vi "DB Driver Main.vi"(0 "Table /DBName/Query":string="KMP", 1 "Option":T1, 2 "Database Name":string="MISPLDBSK06", 5 "Column Names":string[](array[string]), 9 "DB Connection Details":cluster{"UserID":string, "Password":string}={"UserID"="sa", "Password"="12345"}, 11 "error in":errorcluster, 12 "Where":string, 13 "Workstation ID/ Pc Name":string="MISPLDBSK06", 14 "Order By":string) -> (3 "Record Affected":i32, 4 "ADODB._Connection":refnum<k7>, 6 "Selected Data":string[][](array[string]), 10 "element":string, 15 "error out":errorcluster)   [LabVIEW 2017]
uses:
  DB Driver Main Options.ctl
panel:
  out "No.of Row":i32
  # "Output"
  # "Input"
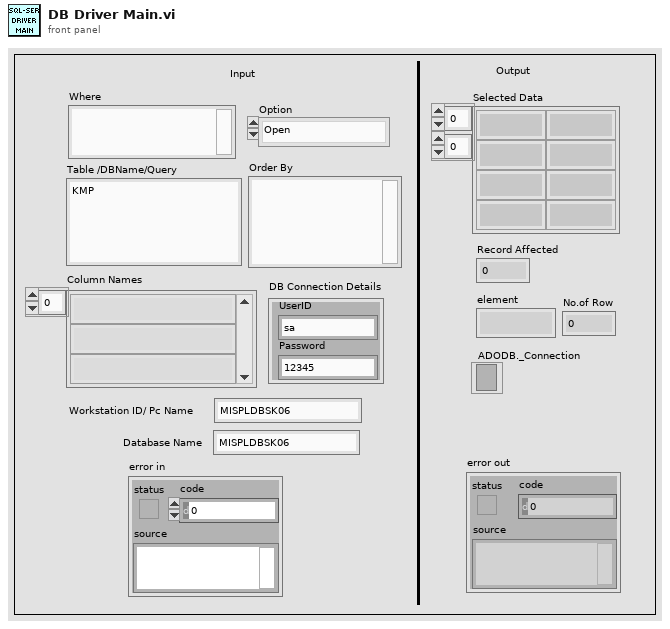
[diagram p1: front panel]
types:
  T1 = typedef "DB Driver Main Options.ctl" = enum16{"Open", "RefOut", "Select", "Execute", "Update", "Insert 2D", "Insert OrUpdate", "Close"}
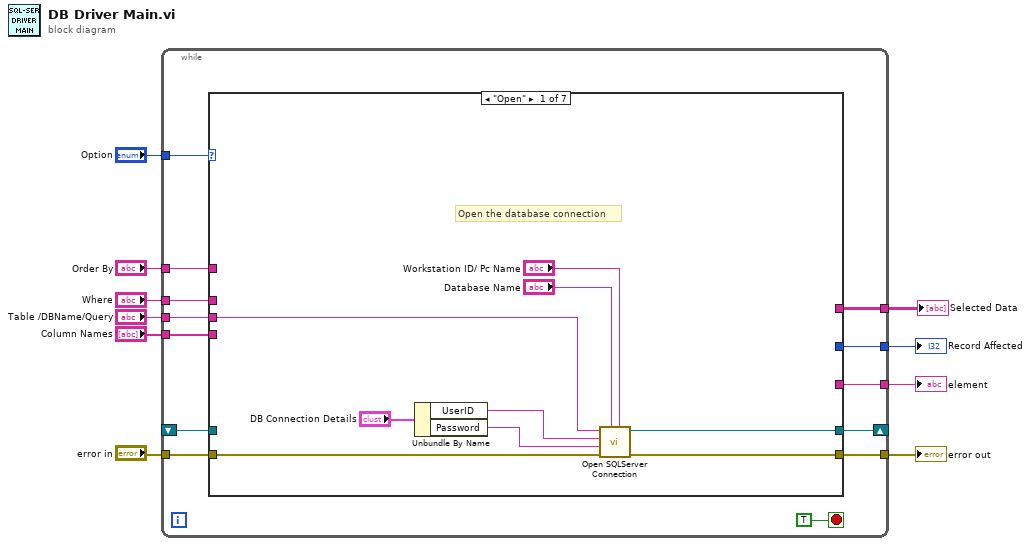
[diagram p0: block diagram]
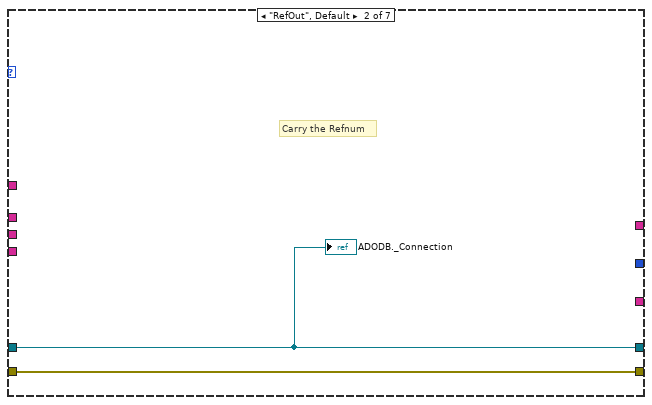
[diagram p2: hidden frame]
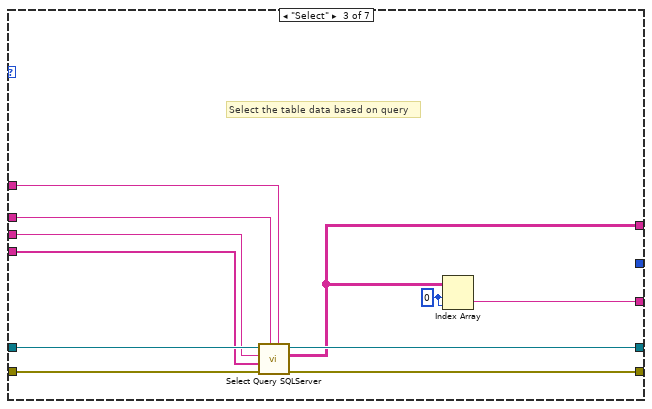
[diagram p3: hidden frame]
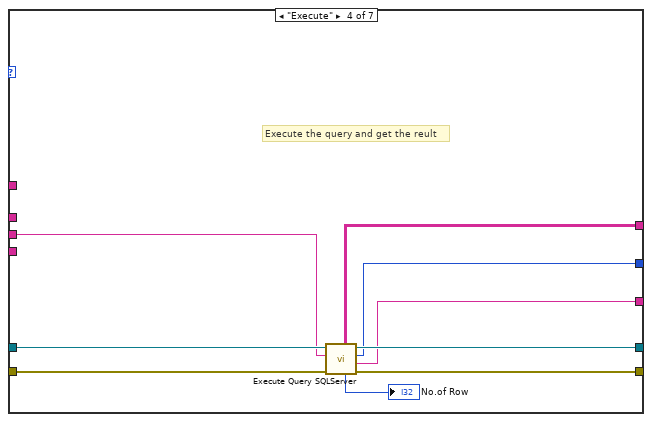
[diagram p4: hidden frame]
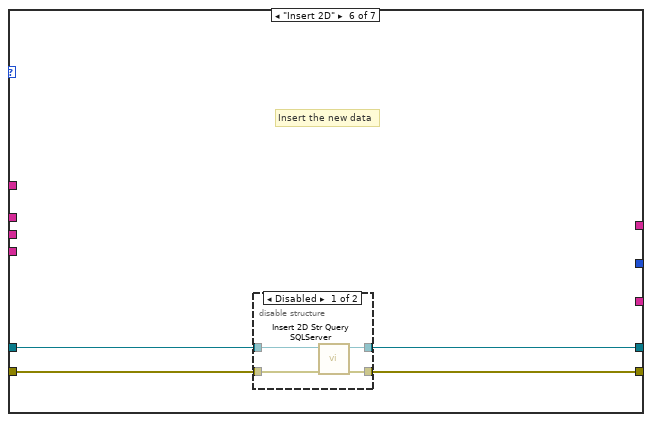
[diagram p6: hidden frame]
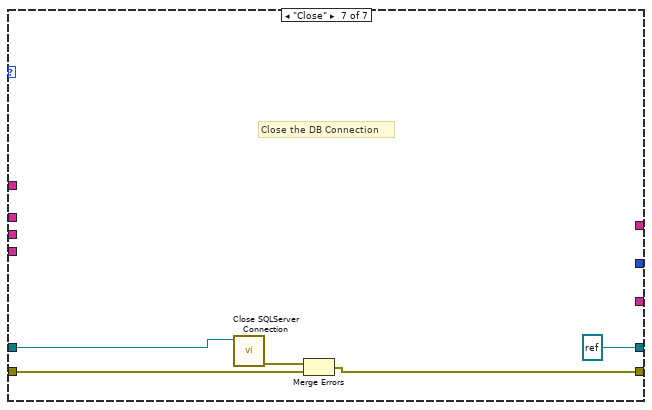
[diagram p8: hidden frame]
diagram:
  n1 = while {
    tunnel: "Option" -> [w22]
    tunnel: "error in" -> [w21]
    tunnel: [w20] -> w8
    shift-right: [w19] -> _
    shift-left: _ -> [w18]
    tunnel: "Where" -> [w17]
    tunnel: "Table /DBName/Query" -> [w16]
    tunnel: "Column Names" -> [w15]
    tunnel: [w14] -> w5
    tunnel: "Order By" -> [w13]
    tunnel: [w12] -> w2
    tunnel: [w11] -> w1
    stop <- TRUE stop-if-true
    n2 = case shown="\"Open\"" w22 {
      tunnel: w21 -> [w32 w34 w43 w54 w55 w58 w69]
      tunnel: [w31 w34 w42 w53 w55 w57 w68] -> w20
      tunnel: [w30 w33 w44 w51 w56 w59 refnum<k7> refnum ("ADODB._Connection")] -> w19
      tunnel: w18 -> [_ w33 w45 w52 w56 w60 w71]
      tunnel: w17 -> [_ _ w41 _ _ _ _]
      tunnel: w16 -> [w29 _ w40 w50 _ _ _]
      tunnel: w15 -> [_ _ w39 _ _ _ _]
      tunnel: [_ _ w37 w49 _ _ _] -> w14
      tunnel: w13 -> [_ _ w38 _ _ _ _]
      tunnel: [_ _ _ w48 _ _ _] -> w12
      tunnel: [_ _ w35 w47 _ _ _] -> w11
      frame "Open" {
        # "Open the database connection"
        n3 = Unbundle By Name("DB Connection Details") -> ("UserID"=w25:string, "Password"=w24:string)
        n4 = call "Open SQLServer Connection.vi"("Workstation ID"="Workstation ID/ Pc Name", "Data Source"="Database Name", "error in (no error)"=w32, "Password"=w24, "UserID"=w25, "DB Name"=w29) -> ("error out"=w31:errorcluster, "ADODB._Connection 2"=w30:refnum<k7>)  [unwired: 4 in]
      }
      frame "RefOut", Default {
        # "Carry the Refnum"
        "ADODB._Connection" <- w33
      }
      frame "Select" {
        w36 = 0 ("index (row)")
        # "Select the table data based on query"
        n5 = call "Select Query SQLServer.vi"("Order By"=w38, "Where"=w41, "error in (no error)"=w43, "Column Names"=w39, "Table Name"=w40, "ADODB._Connection"=w45) -> ("error out"=w42:errorcluster, "Selected Data"=w37:string[][], "ADODB._Connection 2"=w44:refnum<k7>)  [unwired: 2 in, 1 out]
        n6 = Index Array(array=w37, index (row)=w36, index (col)=w36) -> (element=w35:string)
      }
      frame "Execute" {
        # "Execute the query and get the reult"
        n7 = call "Execute Query SQLServer.vi"("error in (no error)"=w54, "Query"=w50, "ADODB._Connection"=w52) -> ("error out"=w53:errorcluster, "element"=w47:string, "Record Affected"=w48:i32, "ADODB._Connection 2"=w51:refnum<k7>, "No.of Row"=→"No.of Row":i32, "Data"=w49:string[][])  [unwired: 3 in]
      }
      frame "Update" {
        # "Update the existing data"
      }
      frame "Insert 2D" {
        # "Insert the new data"
        n8 = disable-structure shown="Disabled" {
          disable-tunnel: w60 -> [w64 w66]
          disable-tunnel: [w63 w66] -> w59
          disable-tunnel: w58 -> [w62 w65]
          disable-tunnel: [w61 w65] -> w57
          frame Disabled {
            n9 = call "Insert 2D Str Query SQLServer.vi"("error in (no error)"=w62, "ADODB._Connection"=w64) -> ("error out"=w61:errorcluster, "ADODB._Connection 2"=w63:refnum<k7>)  [unwired: 7 in, 1 out]
          }
          frame Enabled {
          }
        }
      }
      frame "Close" {
        # "Close the DB Connection"
        n10 = call "Close SQLServer Connection.vi"("ADODB._Connection"=w71) -> ("error out"=w70:errorcluster)  [unwired: 10 in]
        n11 = Merge Errors(w70, w69) -> (w68:errorcluster)
      }
    }
  }
  "error out" <- w8
  "Selected Data" <- w5
  "Record Affected" <- w2
  "element" <- w1
